vi "set variant name.vi"(8 "error in (no error)":errorcluster, 10 "new name":string, 11 "variant in":variant) -> (0 "error out":errorcluster, 3 "variant out":variant)   [LabVIEW 2016, in "JSON Variant Support.lvclass"]
uses:
  JSON Variant Support.lvclass
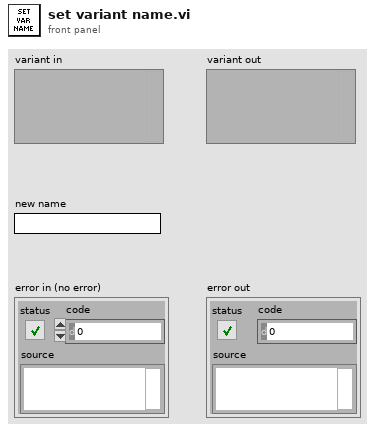
[diagram p1: front panel]
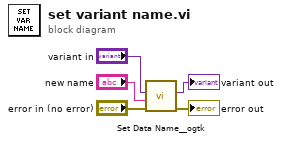
[diagram p0: block diagram]
diagram:
  n1 = call "Set Data Name__ogtk.vi"("error in (no error)"="error in (no error)", "Data Name"="new name", "Data"="variant in") -> ("error out"=→"error out":errorcluster, "Renamed Data"=→"variant out":variant)  [unwired: 7 in]
